vi "RT Driver VI.vi"(6 "Device Clock":string, 9 "Device Inputs FIFO":refnum<k33>, 10 "Device Outputs FIFO":refnum<k33>, 11 "Device Reference":T1 format="%.0x") -> ()   [LabVIEW 2015, in "PXIe 4113 Engine.lvlib"]
uses:
  PXIe 4113 Engine.lvlib
  <vilib>/NI Veristand/Custom Device API/Custom Device Item Ref.ctl
  <vilib>/NI Veristand/Custom Device API/Custom Device Channel Type.ctl
  <vilib>/NI Veristand/Custom Device API/Custom Device API.lvlib
  <vilib>/NI Veristand/Custom Device Tools/Custom Device Utility Library/Custom Device Utility Library.lvlib
panel:
  in  "Initialization Status Notifier":refnum<notifier>
  in  "Status Notifier":refnum<notifier>
  # "Custom Device Template\nv1.0"
  # "Use this template as a starting point for creating a custom device code module. The input controls shown here are specially named controls that the system will use to provide the device loop with data. The controls are not required for the device loop to run. For instance, if the device doesn't produce any output data, then you don't need the Device Outputs FIFO control. If you do use these controls, however, they need to have these exact names to be functional."
  # "The optional status notifier element is used to notify the RT engine of the last state of the custom device, and to indicate the device has completed execution. If this control is not used, a default No Error value is returned to the system when the device finishes execution.\n\nNote: This error state is not checked until the system shuts down. Use an output status channel to send more immediate status values to the system."
  # "This optional input can be used to send the VeriStand Engine the final status of the custom device initalization process. If this control exists on the custom device front panel, the VeriStand Engine will wait for a status update before starting up. If the custom device reports an error, that will abort the execution of the current configuration in the VeriStand Engine.\n\nThis control can be deleted if the custom device does not need to send the initialization status update."
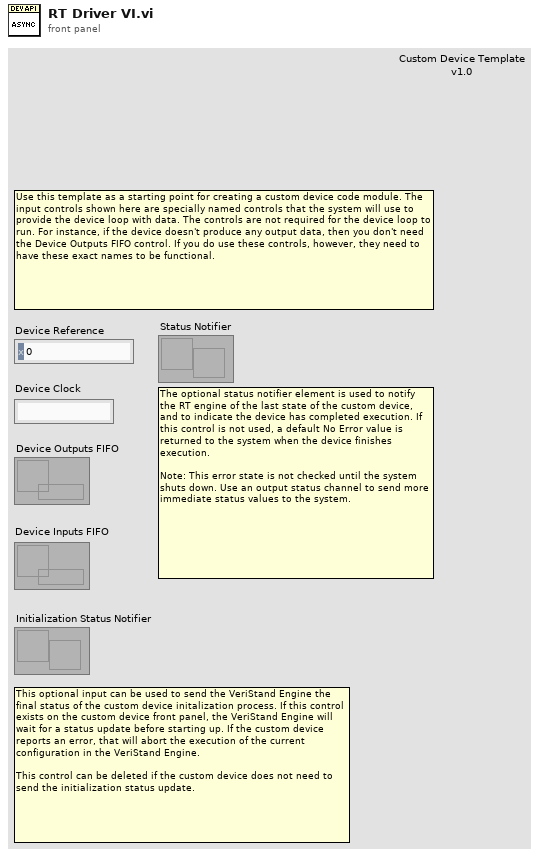
[diagram p1: front panel]
types:
  T1 = typedef "Custom Device API.lvlib/Custom Device Item Ref.ctl" = u64
  T2 = typedef "Custom Device API.lvlib/Custom Device Channel Type.ctl" = enum16{"Input", "Output"}
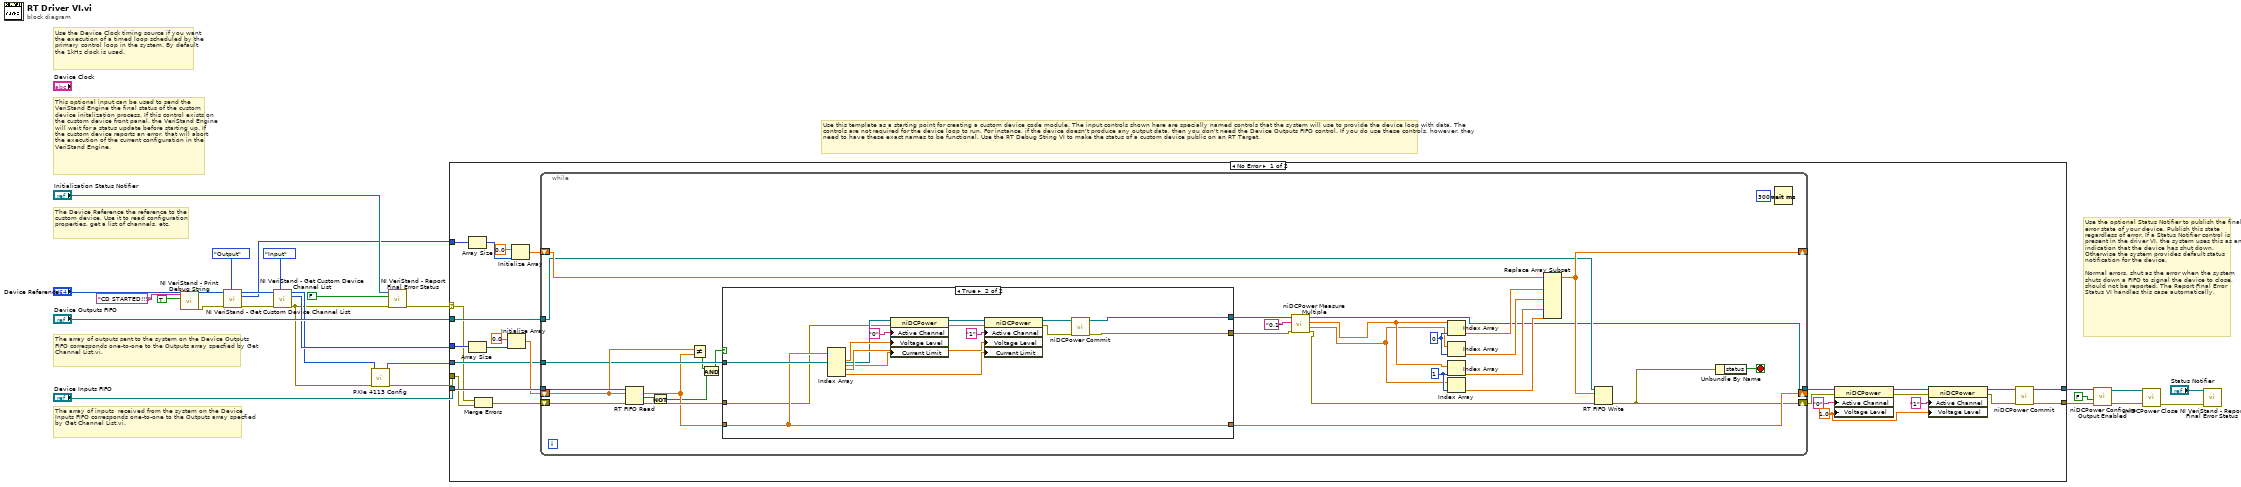
[diagram p0: block diagram]
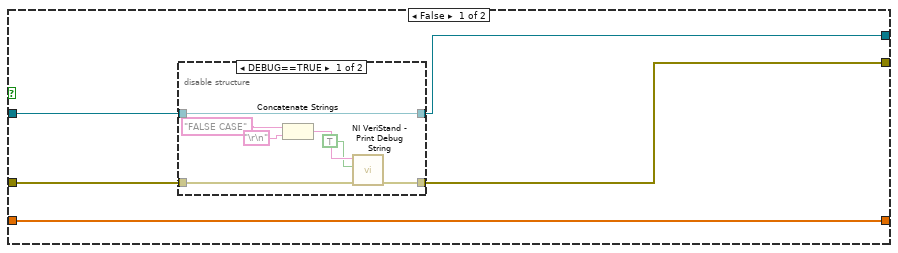
[diagram p2: hidden frame]
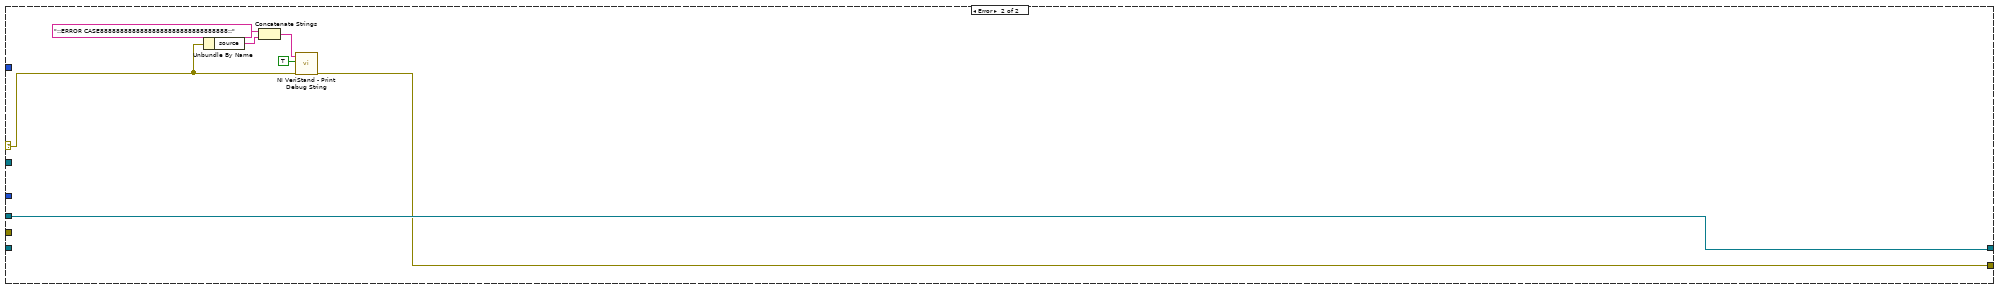
[diagram p4: hidden frame]
diagram:
  # "This optional input can be used to send the VeriStand Engine the final status of the custom device initalization process. If this control exists on the custom device front panel, the VeriStand Engine will wait for a status update before starting up. If the custom device reports an error, that will abort the execution of the current configuration in the VeriStand Engine."
  # "The array of inputs  received from the system on the Device Inputs FIFO corresponds one-to-one to the Outputs array specfied by Get Channel List.vi."
  # "Use the optional Status Notifier to publish the final error state of your device. Publish this state regardless of error. If a Status Notifier control is present in the driver VI, the system uses this as an indication that the device has shut down. Otherwise the system provides default status notification for the device.\n\nNormal errors, shut as the error when the system shuts down a FIFO to signal the device to close, should not be reported. The Report Final Error Status VI handles this case automatically."
  # "The array of outputs sent to the system on the Device Outputs FIFO corresponds one-to-one to the Outputs array specfied by Get Channel List.vi."
  # "The Device Reference the reference to the custom device. Use it to read configuration properties, get a list of channels, etc."
  # "Use the Device Clock timing source if you want the execution of a timed loop scheduled by the primary control loop in the system. By default the 1kHz clock is used."
  # "Use this template as a starting point for creating a custom device code module. The input controls shown here are specially named controls that the system will use to provide the device loop with data. The controls are not required for the device loop to run. For instance, if the device doesn't produce any output data, then you don't need the Device Outputs FIFO control. If you do use these controls, however, they need to have these exact names to be functional. Use the RT Debug String VI to make the status of a custom device public on an RT Target."
  n1 = call <vilib>:"NI VeriStand - Print Debug String.vi"("Add to log file? (T)"=TRUE, "Message"="CD STARTED!!!!") -> ("error out"=w12:errorcluster)  [unwired: 9 in]
  n2 = call <vilib>:"NI VeriStand - Get Custom Device Channel List.vi"("Channel Type"=Custom_Device_Channel_Type."Output", "error in (no error)"=w12, "Device Ref in"="Device Reference") -> ("error out"=w21:errorcluster, "Specified Channel Ref List"=w18:T1[], "Device Ref out"=w22:T1)  [unwired: 6 out]
  n3 = call <vilib>:"NI VeriStand - Get Custom Device Channel List.vi"("Channel Type"=Custom_Device_Channel_Type."Input", "error in (no error)"=w21, "Device Ref in"=w22) -> ("error out"=w7:errorcluster, "Specified Channel Ref List"=w19:T1[], "Device Ref out"=w14:T1)  [unwired: 6 out]
  n4 = call "PXIe 4113 Config.vi"("error in (no error)"=w7, "Device Ref in"=w14) -> ("error out"=w8:errorcluster, "instrument handle out"=w13:refnum<k15>)  [unwired: 7 in, 1 out]
  n5 = call <vilib>:"NI VeriStand - Report Final Error Status.vi"("error in (no error)"=w7, "Filter FIFO & Shutdown Errors (T)"=FALSE ("Filter FIFO Errors (T)"), "Status Notifier"="Initialization Status Notifier") -> ("error out"=w9:errorcluster)  [unwired: 8 out]
  n6 = case shown="No Error" w9 {
    selector: w9 -> [w40 w113]
    tunnel: "Device Outputs FIFO" -> [w51 _]
    tunnel: "Device Inputs FIFO" -> [w50 _]
    tunnel: w19 -> [w44 _]
    tunnel: w18 -> [w43 _]
    tunnel: [w27 w116] -> w4
    tunnel: w13 -> [w41 w117]
    tunnel: w8 -> [w38 _]
    tunnel: [w30 w117] -> w5
    frame No Error {
      w28 = 1.0 ("Source:DC Voltage:Voltage Level")
      n7 = Array Size(array=w44) -> (size(s)=w42:i32)
      n8 = Array Size(array=w43) -> (size(s)=w45:i32)
      n9 = Merge Errors(w40, w38) -> (w39:errorcluster)
      n10 = Initialize Array(0.0 ("element"), w42) -> (w46:dbl[])
      n11 = Initialize Array(0.0 ("element"), w45) -> (w47:dbl[])
      n12 = while {
        shift-right: [w68] -> _
        shift-left: w46 -> [w73]
        shift-right: [w63] -> w29
        shift-left: w39 -> [w81]
        shift-right: [w79] -> _
        shift-left: w47 -> [w80]
        tunnel: w51 -> [w78]
        tunnel: w50 -> [w77]
        tunnel: w41 -> [w70]
        tunnel: [w57] -> w31
        stop <- w71 stop-if-true
        w74 = 1 ("index")
        w75 = 0 ("index")
        n13 = RT FIFO Read(0:w77, 1:w73, 3:w81) -> (9:w69:dbl[], 10:w56:bool, 11:w72:errorcluster)  [unwired: 3 out]
        n14 = Not(x=w56) -> (.not. x?=w54:bool)
        n15 = Not Equal?(x=w73, y=w69) -> (x != y?=w55:bool)
        n16 = And(x=w55, y=w54) -> (x .and. y?=w53:bool)
        n17 = case shown="True" w53 {
          tunnel: w72 -> [w84 w99]
          tunnel: [w83 w100] -> w61
          tunnel: w70 -> [w85 w105]
          tunnel: w69 -> [w86 w104]
          tunnel: [w86 w104] -> w68
          tunnel: [w82 w98] -> w62
          frame False {
            n18 = disable-structure shown="DEBUG==TRUE" {
              disable-tunnel: w85 -> [w87 w94]
              disable-tunnel: w84 -> [w89 w95]
              disable-tunnel: [w88 w95] -> w83
              disable-tunnel: [w87 w94] -> w82
              frame condition #0 {
                n19 = Concatenate Strings("FALSE CASE" ("Message"), "\r\n") -> (w93:string)
                n20 = call <vilib>:"NI VeriStand - Print Debug String.vi"("error in (no error)"=w89, "Add to log file? (T)"=TRUE, "Message"=w93) -> ("error out"=w88:errorcluster)  [unwired: 8 in]
              }
              frame condition #1 (active) {
              }
            }
          }
          frame True {
            n21 = Index Array(array=w104) -> (element #1=w107:dbl, element #2=w97:dbl, element #3=w106:dbl, element #4=w96:dbl)  [unwired: 4 in]
            n22 = property class="niDCPower"(reference=w105, error in=w99, "Active Channel"="0", "Voltage Level"=w107, "Current Limit"=w97) -> (reference out=w108:refnum<k15>, error out=w103:errorcluster)
            n23 = property class="niDCPower"(reference=w108, error in=w103, "Active Channel"="1", "Voltage Level"=w106, "Current Limit"=w96) -> (reference out=w102:refnum<k15>, error out=w101:errorcluster)
            n24 = call <instrlib>:"niDCPower Commit.vi"("error in (no error)"=w101, "instrument handle"=w102) -> ("error out"=w100:errorcluster, "instrument handle out"=w98:refnum<k15>)  [unwired: 8 in]
          }
        }
        n25 = call <instrlib>:"niDCPower Measure Multiple.vi"("error in (no error)"=w61, "channel name"="0,1", "instrument handle"=w62) -> ("error out"=w60:errorcluster, "current measurements"=w58:dbl[], "voltage measurements"=w59:dbl[], "instrument handle out"=w57:refnum<k15>)  [unwired: 5 in]
        n26 = Index Array(array=w59, index=w75) -> (element=w67:dbl)
        n27 = Index Array(array=w58, index=w75) -> (element=w66:dbl)
        n28 = Index Array(array=w59, index=w74) -> (element=w65:dbl)
        n29 = Index Array(array=w58, index=w74) -> (element=w64:dbl)
        n30 = Replace Array Subset(array=w80, new element #1=w67, new element #2=w66, new element #3=w65, new element #4=w64) -> (w79:dbl[])  [unwired: 4 in]
        n31 = RT FIFO Write(0:w78, 1:w79, 3:w60) -> (11:w63:errorcluster)  [unwired: 1 in, 4 out]
        n32 = Unbundle By Name(w63) -> ("status"=w71:bool)
        n33 = Wait (ms)(milliseconds to wait=u32 300) -> ()  [unwired: 1 out]
      }
      n34 = property class="niDCPower"(reference=w31, error in=w29, "Active Channel"="0", "Voltage Level"=w28) -> (reference out=w35:refnum<k15>, error out=w34:errorcluster)
      n35 = property class="niDCPower"(reference=w35, error in=w34, "Active Channel"="1", "Voltage Level"=w28) -> (reference out=w33:refnum<k15>, error out=w32:errorcluster)
      n36 = call <instrlib>:"niDCPower Commit.vi"("error in (no error)"=w32, "instrument handle"=w33) -> ("error out"=w27:errorcluster, "instrument handle out"=w30:refnum<k15>)  [unwired: 8 in]
    }
    frame Error {
      n37 = Unbundle By Name(w113) -> ("source"=w112:string)
      n38 = Concatenate Strings("::ERROR CASE88888888888888888888888888888888::" ("string"), w112) -> (w111:string)
      n39 = call <vilib>:"NI VeriStand - Print Debug String.vi"("error in (no error)"=w113, "Add to log file? (T)"=TRUE, "Message"=w111) -> ("error out"=w116:errorcluster)  [unwired: 8 in]
    }
  }
  n40 = call <instrlib>:"niDCPower Configure Output Enabled.vi"("error in (no error)"=w4, "output enabled"=FALSE, "instrument handle"=w5) -> ("error out"=w2:errorcluster, "instrument handle out"=w3:refnum<k15>)  [unwired: 7 in]
  n41 = call <instrlib>:"niDCPower Close.vi"("error in (no error)"=w2, "instrument handle"=w3) -> ("error out"=w1:errorcluster)  [unwired: 9 in]
  n42 = call <vilib>:"NI VeriStand - Report Final Error Status.vi"("error in (no error)"=w1, "Status Notifier"="Status Notifier") -> ()  [unwired: 1 in, 9 out]
